vi "Decrement Counter with Load.vi"(8 "DEC?":bool, 10 "Reset?":bool, 11 "Load Value":u16) -> (1 "rollover":bool, 3 "count":u16)   [LabVIEW 2011]
doc: "This counter counts from 0....Rollover and then returns to zero\ne.g., If rollover is 2, counter moves as 0,1,2,0,1,2.....\n\n<Latency> = 1 Tick from Reset"
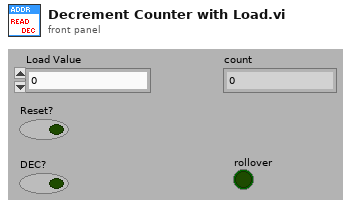
[diagram p1: front panel]
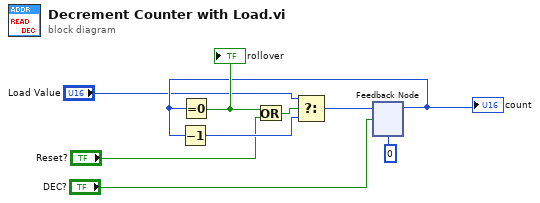
[diagram p0: block diagram]
diagram:
  n1 = feedback #1(u16 0) -> (w2:u16)
  "count" <- w2
  n2 = Decrement(x=w2) -> (x-1=w5:u16)
  n3 = Equal To 0?(x=w2) -> (x = 0?=w8:bool)
  "rollover" <- w8
  n4 = Or(x=w8, y="Reset?") -> (x .or. y?=w7:bool)
  n5 = Select(t="Load Value", s=w7, f=w5) -> (s? t:f=w6:u16)
  n6 = feedback-in #1(w6, "DEC?") -> ()
